vi "modbus-to-real.vi"(8 "error in (no error)":errorcluster, 11 "object in":refnum<class "Type-T-Thermocouple.lvclass">) -> (0 "error out":errorcluster, 3 "object out":refnum<class "Type-T-Thermocouple.lvclass">)   [LabVIEW 2016, in "Type-T-Thermocouple.lvclass"]
doc: "Uses adam formula to convert sensors to real No"
uses:
  Type-T-Thermocouple.lvclass
panel:
  # "Conversion of Modbus reg to a type T thermocouples Degree C"
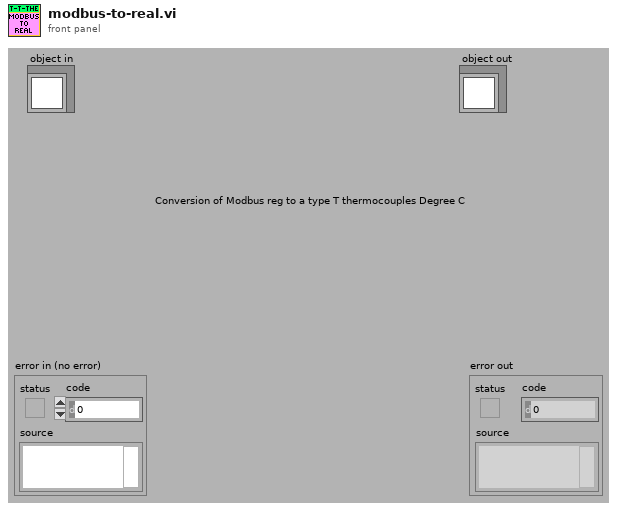
[diagram p1: front panel]
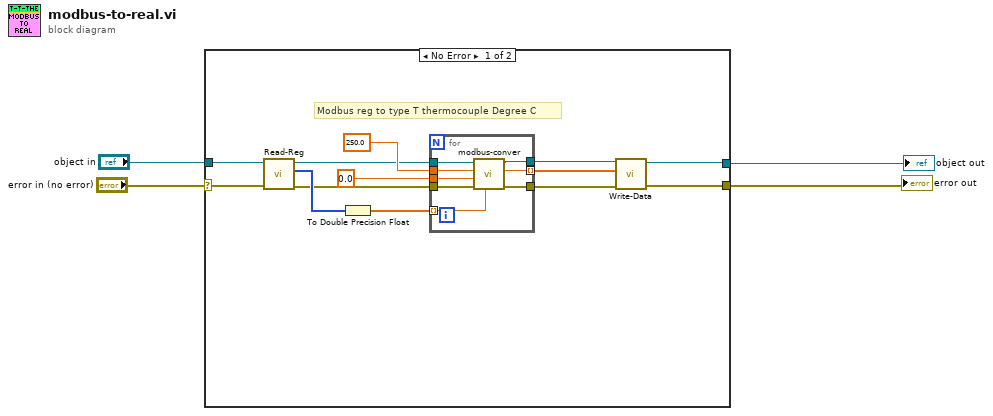
[diagram p0: block diagram]
diagram:
  n1 = case shown="No Error" "error in (no error)" {
    selector: "error in (no error)" -> [w8 w27]
    tunnel: [w12 w27] -> w3
    tunnel: [w15 w26] -> w1
    tunnel: "object in" -> [w11 w26]
    frame No Error {
      # "Modbus reg to type T thermocouple Degree C"
      n2 = call-dynamic "Read-Reg.vi"("error in (no error)"=w8, "Type-K-Thermocouple in"=w11) -> ("error out"=w7:errorcluster, "Modbus-Reg"=w10:u16[], "Type-K-Thermocouple out"=w6:refnum<class "Type-T-Thermocouple.lvclass">)  [unwired: 7 in]
      n3 = To Double Precision Float(number=w10) -> (double precision float=w9:dbl[])
      n4 = for {
        tunnel: w6 -> [w25]
        tunnel: 250.0 ("Scale Max Range") -> [w23]
        tunnel: 0.0 ("Scale Min range") -> [w22]
        tunnel: [w24] -> w13
        tunnel: [w21] -> w14 mode=indexing
        tunnel: w9 -> [w20] mode=indexing
        tunnel: w7 -> [w19]
        tunnel: [w18] -> w5
        n5 = call-dynamic "modbus-conver.vi"("Reg"=w20, "error in (no error)"=w19, "Scale Min range"=w22, "Scale Max Range"=w23, "object in"=w25) -> ("error out"=w24:errorcluster, "output"=w21:dbl, "object out"=w18:refnum<class "Type-T-Thermocouple.lvclass">)  [unwired: 4 in]
      }
      n6 = call-dynamic "Write-Data.vi"("error in (no error)"=w13, "Data"=w14, "Type-K-Thermocouple in"=w5) -> ("error out"=w12:errorcluster, "Type-K-Thermocouple out"=w15:refnum<class "Type-T-Thermocouple.lvclass">)  [unwired: 7 in]
    }
    frame Error {
    }
  }
  "error out" <- w3
  "object out" <- w1
